vi "test-swerve-drive-kinematics-16.vi"() -> (3 "Test Passed":bool)   [LabVIEW 2019]
uses:
  <vilib>/Rock Robotics/WPI/ThirdParty/JAS_Junk/TrajLib/Conv_Deg_Radians.vi
  <vilib>/Rock Robotics/WPI/ThirdParty/JAS_Junk/TrajLib/Rotation2d_CreateAngle.vi
  <vilib>/Rock Robotics/WPI/ThirdParty/JAS_Junk/TrajLib/Trajectory_Library.lvlib
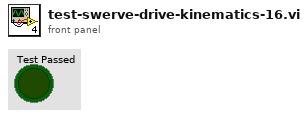
[diagram p1: front panel]
types:
  T1 = typedef "Trajectory_Library.lvlib/ROTATION2D.ctl" = cluster{"VALUE":dbl, "COS":dbl, "SIN":dbl}
  T2 = typedef "Trajectory_Library.lvlib/TRANSLATION2D.ctl" = cluster{"X":dbl, "Y":dbl}
  T3 = typedef "Trajectory_Library.lvlib/SWERVE_DRIVE_MODULE_POSITION.ctl" = cluster{"Distance":dbl, "Angle":T1}
  T4 = typedef "Trajectory_Library.lvlib/SWERVE_DRIVE_KINEMATICS.ctl" = cluster{"NumModules":i32, "InverseKinematics":T5, "ForwardKinematics":T5, "Modules":T2[], "PrevCoR":T2, "SavedModuleStates":T6[]}
  T5 = typedef "NI_Matrix.lvlib/RealMatrix.ctl" = dbl[][]
  T6 = typedef "Trajectory_Library.lvlib/SWERVE_DRIVE_MODULE_STATE.ctl" = cluster{"Speed":dbl, "Angle":T1}
  T7 = typedef "Trajectory_Library.lvlib/TWIST2D.ctl" = cluster{"dX":dbl, "dY":dbl, "dTHETA":dbl}
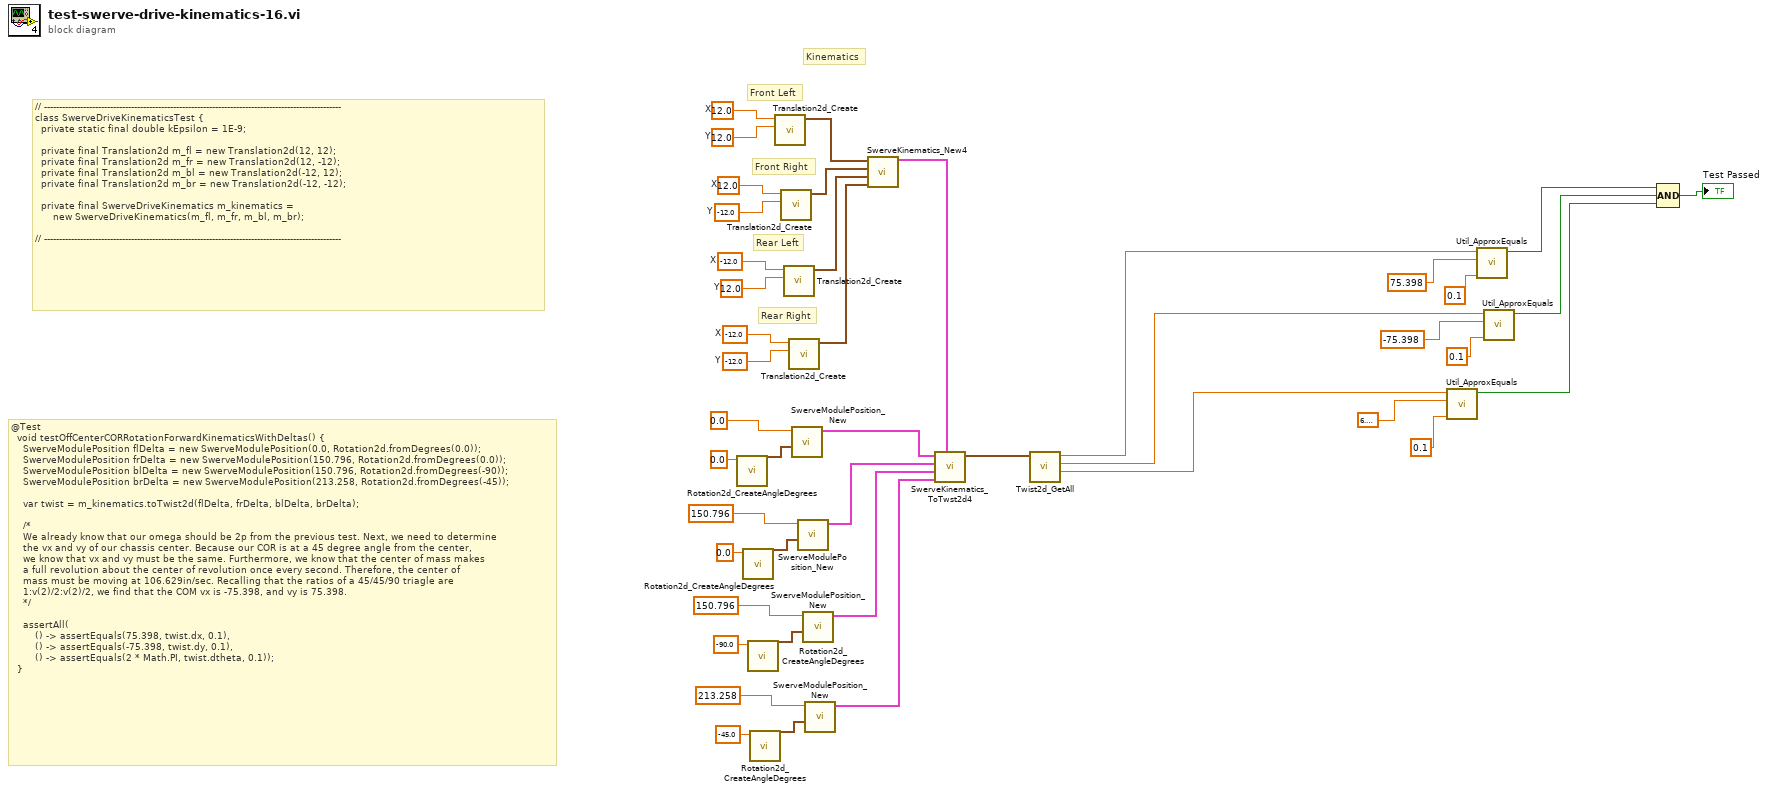
[diagram p0: block diagram]
diagram:
  w39 = -12.0  # X
  w38 = -12.0  # Y
  w37 = -12.0  # X
  w36 = 12.0  # Y
  w35 = 12.0  # X
  w34 = -12.0  # Y
  w33 = 12.0  # X
  w32 = 12.0  # Y
  # "@Test\n  void testOffCenterCORRotationForwardKinematicsWithDeltas() {\n    SwerveModulePosition flDelta = new SwerveModulePosition(0.0, Rotation2d.fromDegrees(0.0));\n    SwerveModulePosition frDelta = new SwerveModulePosition(150.796, Rotation2d.fromDegrees(0.0));\n    SwerveModulePosition blDelta = new SwerveModulePosition(150.796, Rotation2d.fromDegrees(-90));\n    SwerveModulePosition brDelta = new SwerveModulePosition(213.258, Rotation2d.fromDegrees(-45));\n\n    var twist = m_kinematics.toTwist2d(flDelta, frDelta, blDelta, brDelta);\n\n    /*\n    We already know that our omega should be 2p from the previous test. Next, we need to determine\n    the vx and vy of our chassis center. Because our COR is at a 45 degree angle from the center,\n    we know that vx and vy must be the same. Furthermore, we know that the center of mass makes\n    a full revolution about the center of revolution once every second. Therefore, the center of\n    mass must be moving at 106.629in/sec. Recalling that the ratios of a 45/45/90 triagle are\n    1:v(2)/2:v(2)/2, we find that the COM vx is -75.398, and vy is 75.398.\n    */\n\n    assertAll(\n        () -> assertEquals(75.398, twist.dx, 0.1),\n        () -> assertEquals(-75.398, twist.dy, 0.1),\n        () -> assertEquals(2 * Math.PI, twist.dtheta, 0.1));\n  }"
  # "Kinematics"
  # "Rear Right"
  # "Rear Left"
  # "Front Right"
  # "Front Left"
  # "// ---------------------------------------------------------------------------------------------------\nclass SwerveDriveKinematicsTest {\n  private static final double kEpsilon = 1E-9;\n\n  private final Translation2d m_fl = new Translation2d(12, 12);\n  private final Translation2d m_fr = new Translation2d(12, -12);\n  private final Translation2d m_bl = new Translation2d(-12, 12);\n  private final Translation2d m_br = new Translation2d(-12, -12);\n\n  private final SwerveDriveKinematics m_kinematics =\n      new SwerveDriveKinematics(m_fl, m_fr, m_bl, m_br);\n\n// ---------------------------------------------------------------------------------------------------"
  n1 = call <vilib>:"Rotation2d_CreateAngleDegrees.vi"("Angle_Degrees"=0.0) -> ("ROTATION"=w25:T1)  [unwired: 10 in]
  n2 = call <vilib>:"Rotation2d_CreateAngleDegrees.vi"("Angle_Degrees"=0.0) -> ("ROTATION"=w17:T1)  [unwired: 10 in]
  n3 = call <vilib>:"Rotation2d_CreateAngleDegrees.vi"("Angle_Degrees"=-90.0) -> ("ROTATION"=w14:T1)  [unwired: 10 in]
  n4 = call <vilib>:"Rotation2d_CreateAngleDegrees.vi"("Angle_Degrees"=-45.0) -> ("ROTATION"=w11:T1)  [unwired: 10 in]
  n5 = call <vilib>:"Translation2d_Create.vi"("Y"=w32, "X"=w33) -> ("TRANSLATION"=w40:T2)  [unwired: 9 in]
  n6 = call <vilib>:"Translation2d_Create.vi"("Y"=w34, "X"=w35) -> ("TRANSLATION"=w41:T2)  [unwired: 9 in]
  n7 = call <vilib>:"Translation2d_Create.vi"("Y"=w36, "X"=w37) -> ("TRANSLATION"=w42:T2)  [unwired: 9 in]
  n8 = call <vilib>:"Translation2d_Create.vi"("Y"=w38, "X"=w39) -> ("TRANSLATION"=w43:T2)  [unwired: 9 in]
  n9 = call <vilib>:"SwerveModulePosition_New.vi"("ROTATION"=w25, "Distance"=0.0 ("Speed")) -> ("SWERVE_DRIVE_MODULE_POSITION"=w8:T3)  [unwired: 9 in]
  n10 = call <vilib>:"SwerveModulePosition_New.vi"("ROTATION"=w17, "Distance"=150.796 ("Speed")) -> ("SWERVE_DRIVE_MODULE_POSITION"=w7:T3)  [unwired: 9 in]
  n11 = call <vilib>:"SwerveModulePosition_New.vi"("ROTATION"=w14, "Distance"=150.796 ("Speed")) -> ("SWERVE_DRIVE_MODULE_POSITION"=w6:T3)  [unwired: 9 in]
  n12 = call <vilib>:"SwerveModulePosition_New.vi"("ROTATION"=w11, "Distance"=213.258 ("Speed")) -> ("SWERVE_DRIVE_MODULE_POSITION"=w5:T3)  [unwired: 9 in]
  n13 = call <vilib>:"SwerveKinematics_New4.vi"("wheel 3"=w43, "wheel 2"=w42, "wheel 1"=w41, "wheel 0"=w40) -> ("SWERVE_DRIVE_KINEMATICS"=w22:T4)  [unwired: 7 in]
  n14 = call <vilib>:"SwerveKinematics_ToTwst2d4.vi"("in SWERVE_DRIVE_KINEMATICS"=w22, "Wheel Delta 3"=w5, "Wheel Delta 2"=w6, "Wheel Delta 1"=w7, "Wheel Delta 0"=w8) -> ("Twist2d"=w21:T7)  [unwired: 5 in, 1 out]
  n15 = call <vilib>:"Twist2d_GetAll.vi"("TWIST"=w21) -> ("dTHETA"=w18:dbl, "dY"=w19:dbl, "dX"=w20:dbl)  [unwired: 8 in]
  n16 = call <vilib>:"Util_ApproxEquals.vi"("Tolerance"=0.1, "Value 2"=6.283185307179586, "Value 1"=w18) -> ("ApproxEquals"=w27:bool)  [unwired: 8 in]
  n17 = call <vilib>:"Util_ApproxEquals.vi"("Tolerance"=0.1, "Value 2"=75.398, "Value 1"=w20) -> ("ApproxEquals"=w29:bool)  [unwired: 8 in]
  n18 = call <vilib>:"Util_ApproxEquals.vi"("Tolerance"=0.1, "Value 2"=-75.398, "Value 1"=w19) -> ("ApproxEquals"=w28:bool)  [unwired: 8 in]
  n19 = Compound Arithmetic op=AND(w29, w28, w27) -> (→"Test Passed":bool)
